vi "界面UI.vi"() -> ()   [LabVIEW 2016, in "超标留样集成.lvlib"]
uses:
  DR803M4/Vis/Global variable/input variable.vi
  <vilib>/Utility/config.llb/NI_LVConfig.lvlib
  DR803M4/DR803M4.lvlib
panel:
  in  "超标浓度":bool
  in  "修改超标留样型号":bool
  out "x=y?":bool
  in  "锁":bool
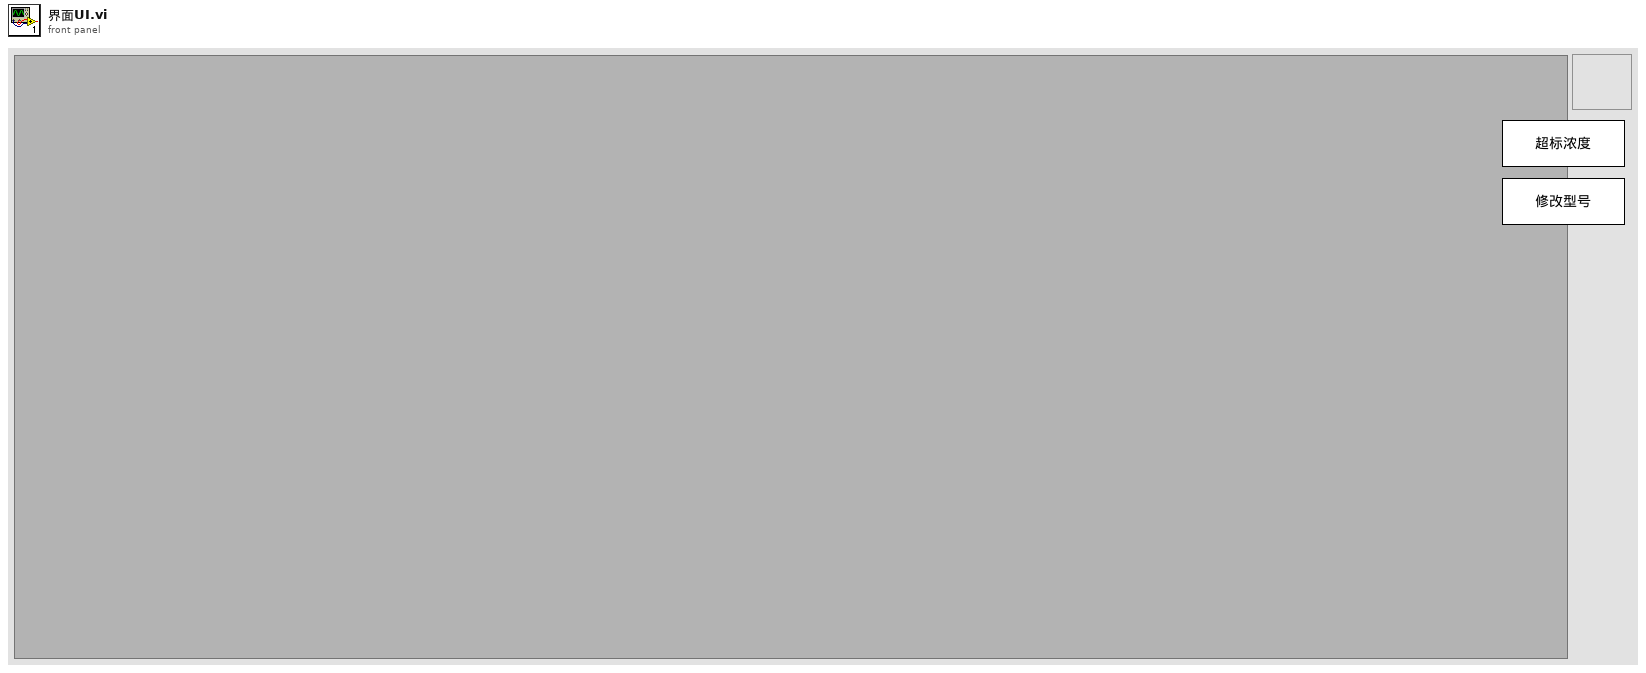
[diagram p1: front panel]
types:
  T1 = typedef "超标留样交互.ctl" = cluster{"当前瓶号":u16}
  T2 = typedef "NI_LVConfig.lvlib/Config Data RefNum.ctl" = refnum<k1>
  T3 = enum16{"德润DR803M", "德润DR803L", "德润DR803F", "科盛超标留样", "德润DR803M4"}
  T4 = enum32{"Bad", "Idle", "Run top level", "Running"}
  T5 = cluster{"仪器时间":timestamp, "工作状态":u16, "工作进程":u16, "采样模式":u16, "采样瓶数":dbl, "当前瓶号":dbl, "设定平行样数":dbl, "已采平行样":dbl, "设定每瓶采样次数":dbl, "已采次数":dbl, "当前瓶采样量":dbl, "瞬时流量":dbl, "累积流量":dbl, "混匀桶已采次数":dbl, "COD":dbl, "NH3N":dbl, "门状态":u16, "采样泵使能":dbl, "采样泵方向":dbl, "导流电机使能":dbl, "导流电机方向":dbl, "阀A":dbl, "阀B":dbl, "阀C":dbl, "外置泵":dbl, "预留":dbl}
  T6 = cluster{"工作状态":u16, "工作进程":u16, "仪器时间":timestamp, "采样模式":u16, "当前瓶号":dbl, "采样瓶数":dbl, "每瓶采样次数":dbl, "当前瓶已采次数":dbl, "当前瓶采样量":dbl, "采样量定量":dbl, "采样量比例":dbl, "瞬时流量":dbl, "累积流量":dbl, "外置泵状态":dbl, "采样泵状态":dbl, "采样泵方向":dbl, "采样阀":dbl, "采样瓶转盘":dbl, "排水阀":dbl, "清洗泵":dbl, "清洗管工作":dbl, "清洗管电源":dbl, "清洗管运行方向":dbl, "门状态":u16, "采水管有水检测":dbl}
  T7 = cluster{"远程留样":u16, "门禁标志":u16, "门禁密码":u32, "采样器进程":u16, "版本号":string, "启停":u16, "当前瓶号":u16, "采样模式选择":u16, "单次采样量":u16, "时间间隔":u16}
  T8 = cluster{"确定":bool, "单选按钮":enum32{"德润DR803M", "德润DR803L", "德润DR803F", "科盛超标留样", "德润DR803M4"}}
  T9 = enum32{"德润DR803M", "德润DR803L", "德润DR803F", "科盛超标留样", "德润DR803M4"}
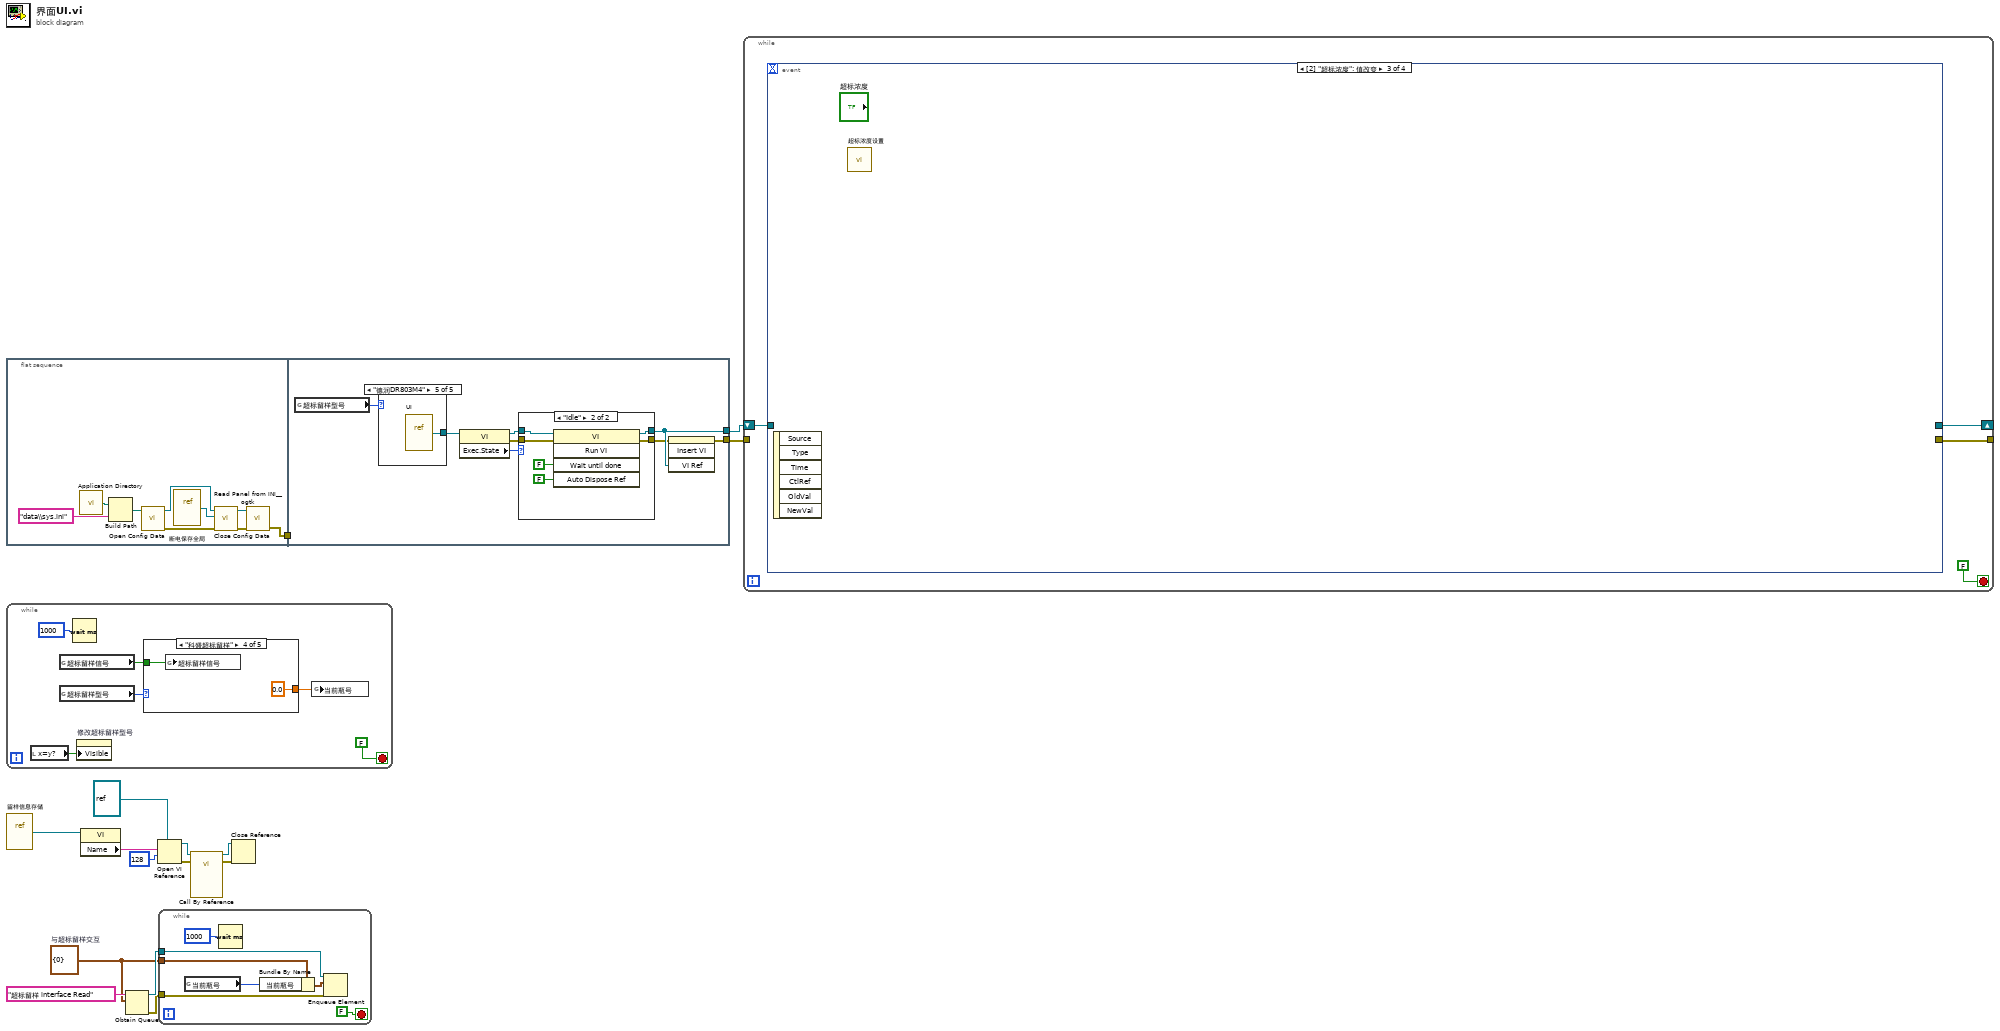
[diagram p0: block diagram]
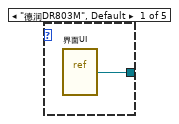
[diagram p2: hidden frame]
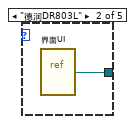
[diagram p3: hidden frame]
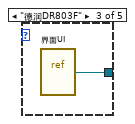
[diagram p4: hidden frame]
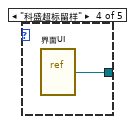
[diagram p5: hidden frame]
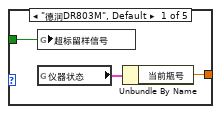
[diagram p7: hidden frame]
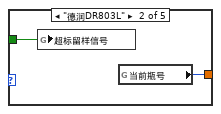
[diagram p8: hidden frame]
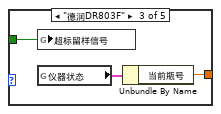
[diagram p9: hidden frame]
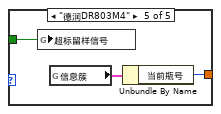
[diagram p10: hidden frame]
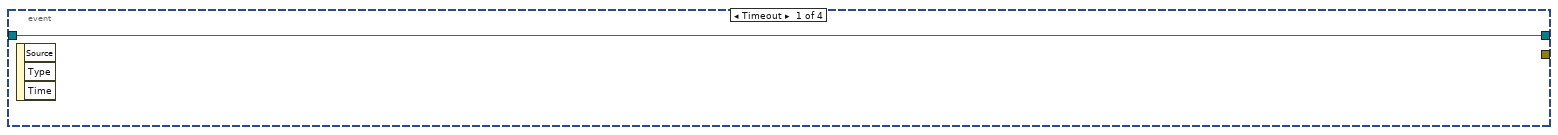
[diagram p11: hidden frame]
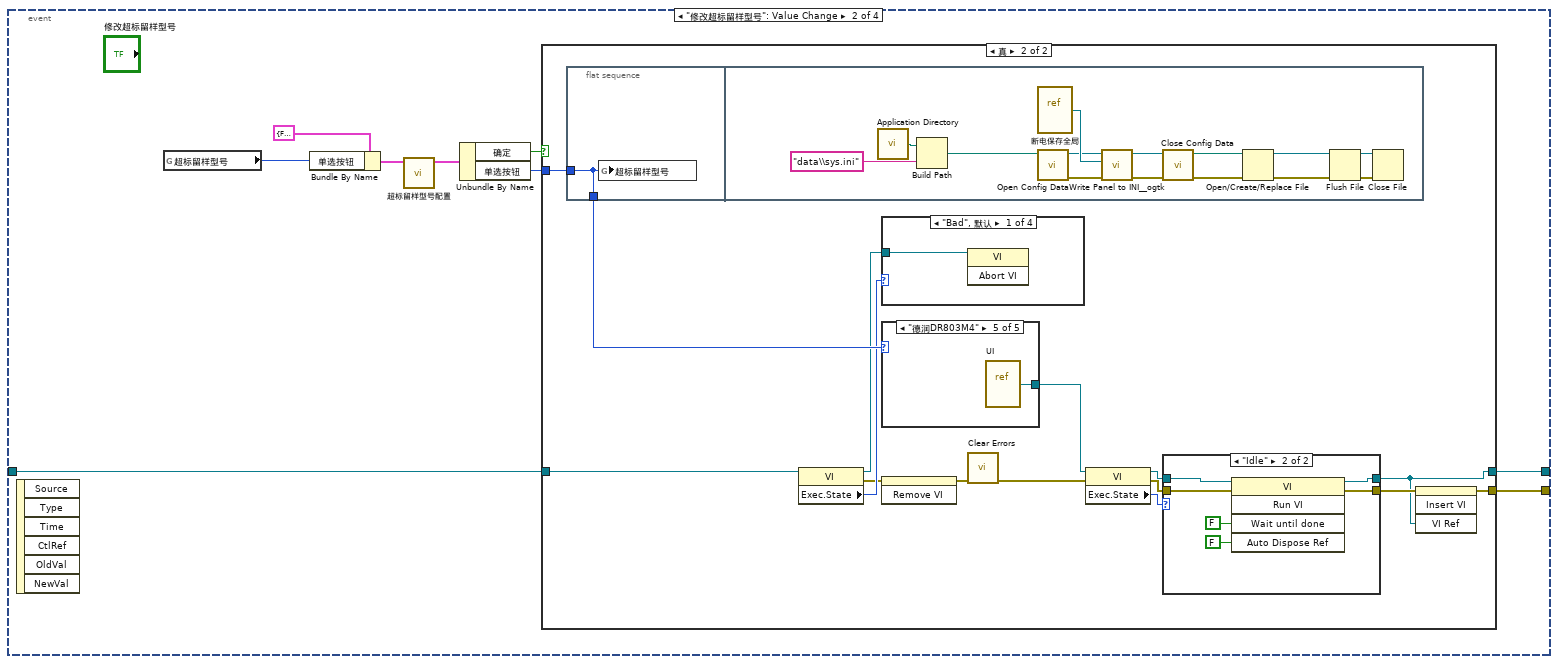
[diagram p12: hidden frame]
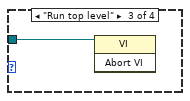
[diagram p15: hidden frame]
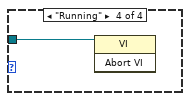
[diagram p16: hidden frame]
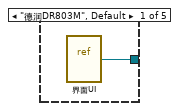
[diagram p17: hidden frame]
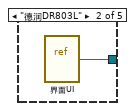
[diagram p18: hidden frame]
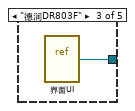
[diagram p19: hidden frame]
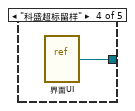
[diagram p20: hidden frame]
diagram:
  w1 = T1 {"当前瓶号"=0}  # 与超标留样交互
  n1 = flat-sequence {
    tunnel: [w16] -> w13
    tunnel: [w27] -> w15
    tunnel: [w25] -> w14
    tunnel: w13 -> [_]
    frame #0 {
      n2 = call <vilib>:"Application Directory.vi"() -> ("Application Directory"=w17:path)
      n3 = Build Path(base path=w17, name or relative path="data\\sys.ini" ("名称或相对路径")) -> (appended path=w19:path)
      n4 = call <vilib>:"Open Config Data.vi"("configuration file path"=w19) -> ("error out"=w23:errorcluster, "refnum"=w20:T2)  [unwired: 8 in, 1 out]
      n5 = vi-ref "断电保存全局.vi"() -> (w21:refnum<vi>)
      n6 = call <userlib>:"Read Panel from INI__ogtk.vi"("error in (no error)"=w23, "VI ref"=w21, "refnum"=w20) -> ("error out"=w24:errorcluster, "refnum out"=w22:T2)  [unwired: 7 in]
      n7 = call <vilib>:"Close Config Data.vi"("error in (no error)"=w24, "refnum"=w22) -> ("error out"=w16:errorcluster)  [unwired: 8 in, 1 out]
    }
    frame #1 {
      n8 = global read "断电保存全局.vi" "超标留样型号"() -> (w28:T3)
      n9 = case shown="\"德润DR803M4\"" w28 {
        tunnel: [w33 w34 w35 w36 w37] -> w29
        frame "德润DR803M", Default {
          n10 = vi-ref "界面UI.vi"() -> (w33:refnum<vi>)
        }
        frame "德润DR803L" {
          n11 = vi-ref "界面UI.vi"() -> (w34:refnum<vi>)
        }
        frame "德润DR803F" {
          n12 = vi-ref "界面UI.vi"() -> (w35:refnum<vi>)
        }
        frame "科盛超标留样" {
          n13 = vi-ref "界面UI.vi"() -> (w36:refnum<vi>)
        }
        frame "德润DR803M4" {
          n14 = vi-ref "UI.vi"() -> (w37:refnum<vi>)
        }
      }
      n15 = property class="VI"(reference=w29) -> (reference out=w31:refnum<vi>, error out=w30:errorcluster, "Exec.State"=w32:T4)  [unwired: 1 in]
      n16 = case shown="\"Idle\"" w32 {
        tunnel: w31 -> [w39 w45]
        tunnel: [w39 w42] -> w27
        tunnel: w30 -> [w38 w41]
        tunnel: [w38 w40] -> w26
        frame "Bad", Default {
        }
        frame "Idle" {
          n17 = invoke class="VI" method="Run VI"(reference=w45, error in=w41, "Wait until done"=FALSE ("结束前等待"), "Auto Dispose Ref"=FALSE ("自动销毁引用")) -> (reference out=w42:refnum<vi>, error out=w40:errorcluster)  [unwired: 1 in, 3 out]
        }
      }
      n18 = invoke class="SubPnl" method="Insert VI"(error in=w26, "VI Ref"=w27) -> (error out=w25:errorcluster)  [unwired: 2 in, 3 out]
    }
  }
  n19 = while {
    stop <- FALSE stop-if-true
    n20 = local read "x=y?"() -> (w47:bool)
    n21 = global read "外部交互全局.vi" "超标留样信号"() -> (w48:bool)
    n22 = global read "断电保存全局.vi" "超标留样型号"() -> (w49:T3)
    n23 = Wait (ms)(milliseconds to wait=u32 1000 ("等待时间（毫秒）")) -> ()  [unwired: 1 out]
    n24 = property on="修改超标留样型号" class="Bool"("Visible"=w47) -> ()  [unwired: 2 in, 2 out]
    n25 = case shown="\"科盛超标留样\"" w49 {
      tunnel: w48 -> [w54 w56 w59 w61 w64]
      tunnel: [w52 w55 w57 0.0 ("当前瓶号") w62] -> w46
      frame "德润DR803M", Default {
        n26 = global write "超标留样全局.vi" "超标留样信号"(w54) -> ()
        n27 = global read "超标留样全局.vi" "仪器状态"() -> (w53:T5)
        n28 = Unbundle By Name(w53) -> ("当前瓶号"=w52:dbl)
      }
      frame "德润DR803L" {
        n29 = global write "串口参数断电保存全局变量.vi" "超标留样信号"(w56) -> ()
        n30 = global read "超标留样全局.vi" "当前瓶号"() -> (w55:u16)
      }
      frame "德润DR803F" {
        n31 = global write "超标留样全局.vi" "超标留样信号"(w59) -> ()
        n32 = global read "超标留样全局.vi" "仪器状态"() -> (w58:T6)
        n33 = Unbundle By Name(w58) -> ("当前瓶号"=w57:dbl)
      }
      frame "科盛超标留样" {
        n34 = global write "超标留样全局.vi" "超标留样信号"(w61) -> ()
      }
      frame "德润DR803M4" {
        n35 = global write "input variable.vi" "超标留样信号"(w64) -> ()
        n36 = global read "input variable.vi" "信息簇"() -> (w63:T7)
        n37 = Unbundle By Name(w63) -> ("当前瓶号"=w62:u16)
      }
    }
    n38 = global write "外部交互全局.vi" "当前瓶号"(w46) -> ()
  }
  n39 = vi-ref "留样信息存储.vi"() -> (w12:refnum<vi>)
  n40 = property class="VI"(reference=w12) -> ("Name"=w11:string)  [unwired: 1 in, 2 out]
  n41 = Obtain Queue(name (unnamed)="超标留样 interface Read" ("写入方名称"), element data type=w1) -> (queue out=w4:refnum<queue>, error out=w3:errorcluster)  [unwired: 3 in, 1 out]
  n42 = Open VI Reference(type specifier VI Refnum (for type only)=refnum<vi> refnum, vi path=w11, options=128 ("选项")) -> (vi reference=w9:refnum<vi>, error out=w7:errorcluster)  [unwired: 3 in]
  n43 = while {
    tunnel: w4 -> [w69]
    tunnel: w3 -> [w68]
    tunnel: w1 -> [w67]
    stop <- FALSE stop-if-true
    n44 = global read "外部交互全局.vi" "当前瓶号"() -> (w66:u16)
    n45 = Wait (ms)(milliseconds to wait=u32 1000 ("等待时间（毫秒）")) -> ()  [unwired: 1 out]
    n46 = Bundle By Name(cluster=w67, "当前瓶号"=w66) -> (w65:T1)
    n47 = Enqueue Element(queue=w69, element=w65, error in (no error)=w68) -> ()  [unwired: 1 in, 3 out]
  }
  n48 = call-by-ref "?"(reference=w9, error in=w7) -> (reference out=w5:refnum<vi>, error out=w6:errorcluster)  [unwired: 12 in]
  n49 = Close Reference(reference=w5, error in (no error)=w6) -> ()  [unwired: 1 out]
  n50 = while {
    tunnel: [w75] -> _
    tunnel: w14 -> [_]
    shift-right: [w73] -> _
    shift-left: w15 -> [w72]
    stop <- FALSE stop-if-true
    n51 = event shown="[2] \"超标浓度\": 值改变" {
      selector: _ -> [_ _ _ _]
      dyn-events: _ -> [_ _ _ _]
      timeout: _ -> [_ _ _ _]
      tunnel: [_ w81 _ _] -> w75
      tunnel: [w76 w80 _ _] -> w73
      tunnel: w72 -> [w76 w79 _ _]
      event Timeout {
        n52 = event-data() -> ()  [unwired: 1 in, 3 out]
      }
      event "修改超标留样型号": Value Change {
        n53 = event-data() -> ()  [unwired: 1 in, 6 out]
        n54 = global read "断电保存全局.vi" "超标留样型号"() -> (w85:T3)
        n55 = Bundle By Name(cluster=T8 {"确定"=FALSE, "单选按钮"=enum."德润DR803F"} ("输入"), "单选按钮"=w85) -> (w77:T8)
        n56 = call "超标留样型号配置.vi"("输入"=w77) -> ("输出"=w84:T8)  [unwired: 10 in]
        n57 = Unbundle By Name(w84) -> ("确定"=w82:bool, "单选按钮"=w83:T9)
        n58 = case shown="真" w82 {
          tunnel: w83 -> [_ w101]
          tunnel: [_ w90] -> w81
          tunnel: [w86 w91] -> w80
          tunnel: w79 -> [w86 w95]
          frame False {
          }
          frame True {
            n59 = flat-sequence {
              tunnel: w101 -> [w118]
              tunnel: [w118] -> w96
              frame #0 {
                n60 = global write "断电保存全局.vi" "超标留样型号"(w118) -> ()
              }
              frame #1 {
                n61 = call <vilib>:"Application Directory.vi"() -> ("Application Directory"=w120:path)
                n62 = Build Path(base path=w120, name or relative path="data\\sys.ini" ("名称或相对路径")) -> (appended path=w121:path)
                n63 = vi-ref "断电保存全局.vi"() -> (w123:refnum<vi>)
                n64 = call <vilib>:"Open Config Data.vi"("configuration file path"=w121) -> ("error out"=w125:errorcluster, "refnum"=w122:T2)  [unwired: 8 in, 1 out]
                n65 = call <userlib>:"Write Panel to INI__ogtk.vi"("error in (no error)"=w125, "VI ref"=w123, "refnum"=w122) -> ("error out"=w126:errorcluster, "refnum out"=w124:T2)  [unwired: 7 in]
                n66 = call <vilib>:"Close Config Data.vi"("error in (no error)"=w126, "refnum"=w124) -> ("error out"=w131:errorcluster, "file path"=w132:path)  [unwired: 8 in]
                n67 = Open/Create/Replace File(file path (use dialog)=w132, error in=w131) -> (refnum out=w128:refnum<file>, error out=w127:errorcluster)  [unwired: 4 in, 1 out]
                n68 = Flush File(refnum=w128, error in=w127) -> (refnum out=w129:refnum<file>, error out=w130:errorcluster)
                n69 = Close File(refnum=w129, error in=w130) -> ()  [unwired: 2 out]
              }
            }
            n70 = property class="VI"(reference=w95) -> (reference out=w93:refnum<vi>, error out=w89:errorcluster, "Exec.State"=w94:T4)  [unwired: 1 in]
            n71 = case shown="\"Bad\", 默认" w94 {
              tunnel: w93 -> [w102 _ w103 w104]
              frame "Bad", Default {
                n72 = invoke class="VI" method="Abort VI"(reference=w102) -> ()  [unwired: 2 in, 3 out]
              }
              frame "Idle" {
              }
              frame "Run top level" {
                n73 = invoke class="VI" method="Abort VI"(reference=w103) -> ()  [unwired: 2 in, 3 out]
              }
              frame "Running" {
                n74 = invoke class="VI" method="Abort VI"(reference=w104) -> ()  [unwired: 2 in, 3 out]
              }
            }
            n75 = case shown="\"德润DR803M4\"" w96 {
              tunnel: [w105 w106 w107 w108 w109] -> w97
              frame "德润DR803M", Default {
                n76 = vi-ref "界面UI.vi"() -> (w105:refnum<vi>)
              }
              frame "德润DR803L" {
                n77 = vi-ref "界面UI.vi"() -> (w106:refnum<vi>)
              }
              frame "德润DR803F" {
                n78 = vi-ref "界面UI.vi"() -> (w107:refnum<vi>)
              }
              frame "科盛超标留样" {
                n79 = vi-ref "界面UI.vi"() -> (w108:refnum<vi>)
              }
              frame "德润DR803M4" {
                n80 = vi-ref "UI.vi"() -> (w109:refnum<vi>)
              }
            }
            n81 = invoke class="SubPnl" method="Remove VI"(error in=w89) -> (error out=w88:errorcluster)  [unwired: 2 in, 2 out]
            n82 = call <vilib>:"Clear Errors.vi"("error in (no error)"=w88) -> ("error out"=w87:errorcluster)  [unwired: 5 in, 1 out]
            n83 = property class="VI"(reference=w97, error in=w87) -> (reference out=w99:refnum<vi>, error out=w98:errorcluster, "Exec.State"=w100:T4)
            n84 = case shown="\"Idle\"" w100 {
              tunnel: w99 -> [w111 w117]
              tunnel: [w111 w114] -> w91
              tunnel: w98 -> [w110 w113]
              tunnel: [w110 w112] -> w92
              frame "Bad", Default {
              }
              frame "Idle" {
                n85 = invoke class="VI" method="Run VI"(reference=w117, error in=w113, "Wait until done"=FALSE ("结束前等待"), "Auto Dispose Ref"=FALSE ("自动销毁引用")) -> (reference out=w114:refnum<vi>, error out=w112:errorcluster)  [unwired: 1 in, 3 out]
              }
            }
            n86 = invoke class="SubPnl" method="Insert VI"(error in=w92, "VI Ref"=w91) -> (error out=w90:errorcluster)  [unwired: 2 in, 3 out]
          }
        }
      }
      event "超标浓度": Value Change {
        n87 = event-data() -> ()  [unwired: 1 in, 6 out]
        n88 = call "超标浓度设置.vi"() -> ()  [unwired: 12 in]
      }
      event "锁": Mouse Down {
        n89 = event-data() -> ("CtlRef"=w134:refnum<vi>)  [unwired: 1 in, 7 out]
        n90 = case shown="真" "锁" {
          tunnel: [w138 w145] -> w136
          tunnel: [w137 w145] -> w135
          frame False {
            n91 = call "数字键盘.vi"() -> ("NewNumber"=w141:sgl)  [unwired: 1 in]
            n92 = Equal?(x=w141, y=sgl 23506.0) -> (x = y?=w139:bool)
            n93 = case shown="真" w139 {
              selector: w139 -> [w142 w144]
              tunnel: [w142 w144] -> w138
              tunnel: [w142 w144] -> w137
              frame False {
                n94 = One Button Dialog(message="密码错误" ("消息")) -> ()  [unwired: 1 in, 1 out]
              }
              frame True {
              }
            }
          }
          frame True {
            w145 = FALSE
          }
        }
        "x=y?" <- w136
        n95 = property class="Bool (严格)"(reference=w134, "Value"=w135) -> ()  [unwired: 1 in, 2 out]
      }
    }
  }
